vi "Returning A Value String.vi"(8 "error in (no error)":errorcluster) -> (0 "error out":errorcluster, 3 "function return":string)   [LabVIEW 2009, in "LabVIEWWrapper_PassingDataSampleDLL.lvlib"]
doc: "char* ReturningAValue_String (void);"
uses:
  LabVIEWWrapper_PassingDataSampleDLL.lvlib
  PassingDataSampleDLL.dll
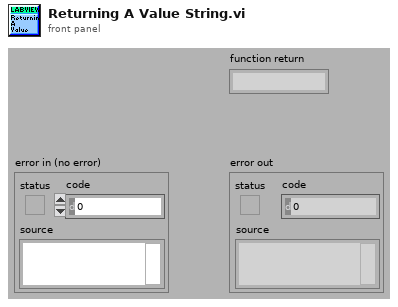
[diagram p1: front panel]
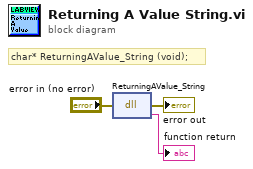
[diagram p0: block diagram]
diagram:
  # "char* ReturningAValue_String (void);"
  n1 = dll-call lib="C:/My Dropbox/Systems Engineering Application/SDK/C Integration/LabVIEWWrapper/PassingDataSampleDLL.*" fn="ReturningAValue_String"(error in="error in (no error)") -> (error out=→"error out":errorcluster, →"function return":string)  [unwired: 2 in, 1 out]
